vi "AssertChannelLoopback.vi"(4 "Tolerance (0.01)":dbl=0.01 format="%#_13g", 6 "Value":dbl, 7 "Timeout (1 second)":dbl=1.0 format="%#_13g", 8 "error in (no error)":errorcluster, 9 "Read Channel":string, 10 "Write Channel":string, 11 "VeriStand Test Case in":refnum<class "VeriStandTestCase.lvclass">) -> (0 "error out":errorcluster, 3 "VeriStand Test Case out":refnum<class "VeriStandTestCase.lvclass">)   [LabVIEW 2027, in "VeriStandTestCase.lvclass"]
uses:
  VeriStandTestCase.lvclass
  VeriStandTestCase.lvclass/VeriStandTestCase.ctl
  VeriStandTestUtilities/VeriStandTestUtilities.lvlib
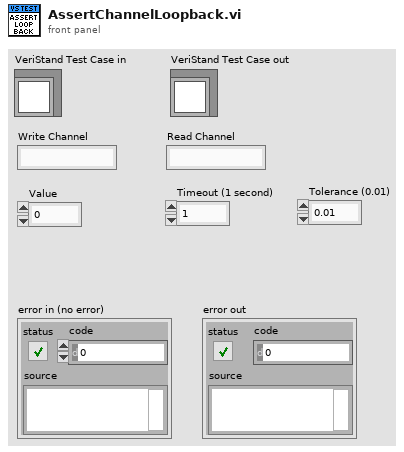
[diagram p1: front panel]
types:
  T1 = typedef "NI_VS Workspace ExecutionAPI.lvlib/WorkspaceAPI.ctl" = refnum<k39>
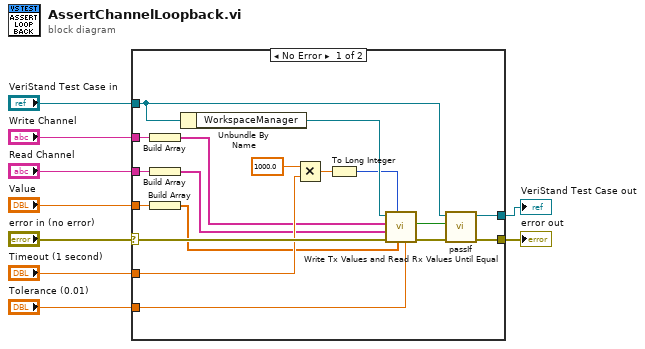
[diagram p0: block diagram]
diagram:
  n1 = case shown="No Error" "error in (no error)" {
    selector: "error in (no error)" -> [w24 w28]
    tunnel: [w27 w28] -> w9
    tunnel: "Read Channel" -> [w16 _]
    tunnel: "Write Channel" -> [w17 _]
    tunnel: "Value" -> [w15 _]
    tunnel: "Timeout (1 second)" -> [w21 _]
    tunnel: "Tolerance (0.01)" -> [w23 _]
    tunnel: "VeriStand Test Case in" -> [w25 w29]
    tunnel: [w26 w29] -> w1
    frame No Error {
      n2 = Build Array(w17) -> (w14:string[])
      n3 = Build Array(w16) -> (w13:string[])
      n4 = Build Array(w15) -> (w12:dbl[])
      n5 = Unbundle By Name(w25) -> ("WorkspaceManager"=w20:T1)
      n6 = Multiply(x=1000.0, y=w21) -> (x*y=w18:dbl)
      n7 = To Long Integer(number=w18) -> (32bit integer=w19:i32)
      n8 = call "Write Tx Values and Read Rx Values Until Equal.vi"("tolerance (0.01)"=w23, "Tx values"=w12, "timeout (1000 ms)"=w19, "error in"=w24, "Rx aliases"=w13, "Tx aliases"=w14, "workspace manager in"=w20) -> ("error out"=w11:errorcluster, "values equal"=w10:bool)  [unwired: 2 in, 1 out]
      n9 = call-dynamic "passIf.vi"("error in (no error)"=w11, "pass"=w10, "TestCase in"=w25) -> ("error out"=w27:errorcluster, "TestCase out"=w26:refnum<class "VeriStandTestCase.lvclass">)  [unwired: 7 in]
    }
    frame Error {
    }
  }
  "error out" <- w9
  "VeriStand Test Case out" <- w1
